vi "Hysteresis-FromFwdBwdHoneyCombStructure.vi"(4 "Max Hysteresis":dbl=0.2 format="%#_13g", 6 "border filter":dbl format="%#_13g", 8 "hypothesis":T1(ring)=enum."middle", 9 "relative Range":dbl=0.5 min=0.0 max=1.0 format="%#_13g", 10 "Pictures":cluster{"Fwd":dbl[][], "Bwd":dbl[][]}) -> (0 "bwd_fwd_weight":cluster{dbl[], dbl[], dbl[]}, 1 "Preisach":dbl[](array[numeric]), 2 "Polynomial Coefficients bwd":dbl[](array[numeric]), 3 "Polynomial Coefficients fwd":dbl[](array[numeric]), 5 "pixel to delete":i32)   [LabVIEW 2016]
uses:
  <vilib>/Analysis/NI_AALPro.lvlib
panel:
  out "Cov processed":dbl[][](graph)
  out "Hysteresis loop":cluster{dbl[], dbl[]}[](graph)
  out "Cov unprocessed":dbl[][](graph)
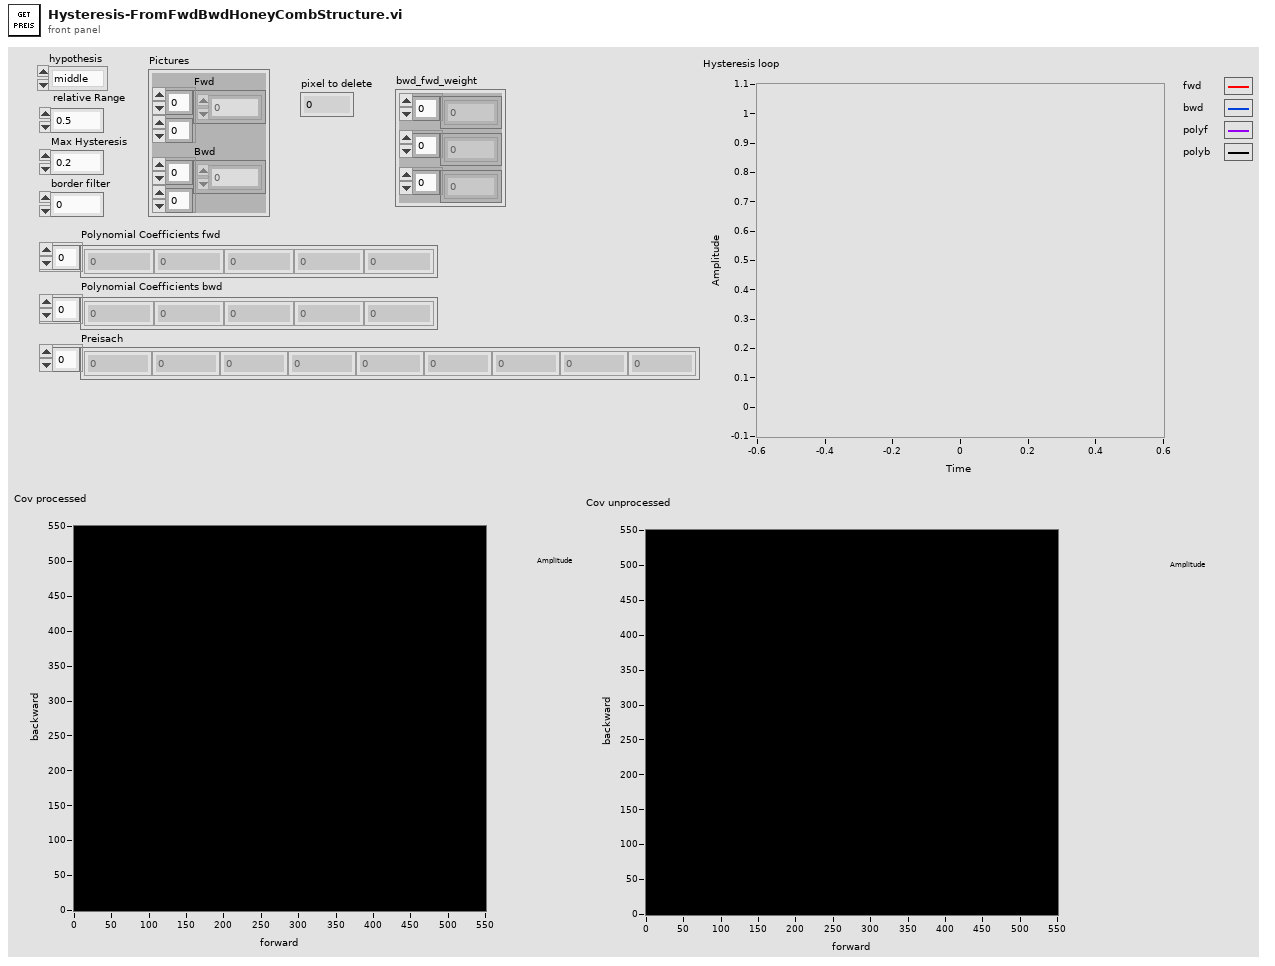
[diagram p1: front panel]
types:
  T1 = enum16{"bwd", "middle", "fwd", "linear", "2nd esti"}
  T2 = cluster{"bwd column corrected":dbl[], "fwd column corrected":dbl[]}
  T3 = cluster{"linear pos ":dbl[], "bwd pos":dbl[], "fwd pos":dbl[]}
  T4 = cluster{"bwd column corrected":dbl[], "fwd column corrected":dbl[], "Values":dbl[]}
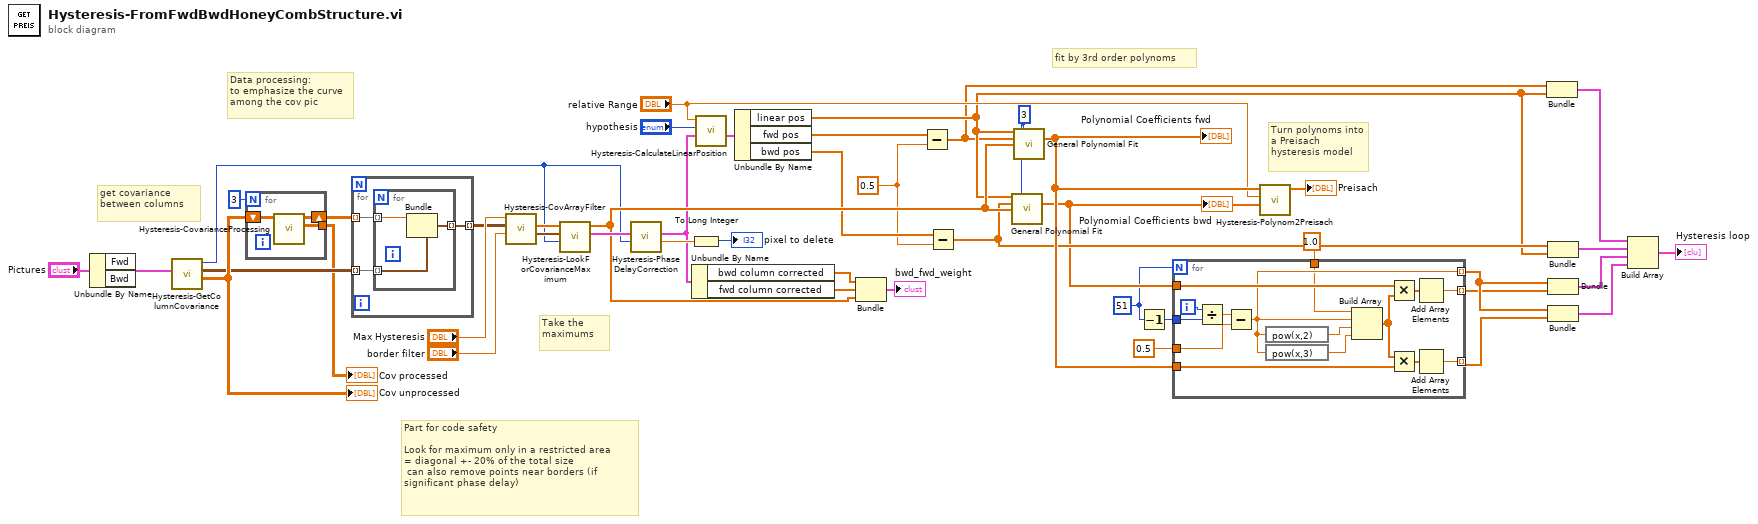
[diagram p0: block diagram]
diagram:
  w7 = 0.5 ("y")
  w4 = 3 ("polynomial order")
  w1 = 51
  # "Take the maximums"
  # "fit by 3rd order polynoms"
  # "Turn polynoms into a Preisach hysteresis model"
  # "Part for code safety\n\nLook for maximum only in a restricted area\n= diagonal +- 20% of the total size\n can also remove points near borders (if significant phase delay)"
  # "Data processing:\nto emphasize the curve\namong the cov pic"
  # "get covariance between columns"
  n1 = Unbundle By Name("Pictures") -> ()  [unwired: 2 out]
  n2 = call "Hysteresis-GetColumnCovariance.vi"("Pictures"="Pictures") -> ("Covariances (2D)"=w32:dbl[][], "Covariances (in cluster)"=w30:cluster{dbl, i32, i32}[][], "Size"=w20:i32)  [unwired: 8 in]
  "Cov unprocessed" <- w32
  n3 = for {
    N: 3 -> [_]
    tunnel: [w46] -> w3
    shift-right: [w47] -> w31
    shift-left: w32 -> [w48]
    n4 = call "Hysteresis-CovarianceProcessing.vi"("Covariances (2D)"=w48) -> ("Covariance Processed (2D)"=w46:dbl[][], "Covariance Data"=w47:dbl[][])  [unwired: 9 in]
  }
  "Cov processed" <- w3
  n5 = for {
    tunnel: w31 -> [w50] mode=indexing
    tunnel: w30 -> [w51] mode=indexing
    tunnel: [w49] -> w29 mode=indexing
    n6 = for {
      tunnel: w51 -> [w54] mode=indexing
      tunnel: w50 -> [w53] mode=indexing
      tunnel: [w52] -> w49 mode=indexing
      n7 = Bundle(cluster=w54, w53) -> (w52:cluster{dbl, i32, i32})  [unwired: 2 in]
    }
  }
  n8 = call "Hysteresis-CovArrayFilter.vi"("filtering"="border filter", "Covariance Corrected"=w29, "Max Hysteresis"="Max Hysteresis") -> ("Cluster filtered"=w41:cluster{dbl, i32, i32}[], "Covariance Values (1D)"=w42:dbl[])  [unwired: 7 in]
  n9 = call "Hysteresis-LookForCovarianceMaximum.vi"("size"=w20, "Cluster filtered"=w41, "Covariance Values (1D)"=w42) -> ("BWD/FWD"=w45:cluster{"bwd column":i32[], "fwd column":i32[]}, "Values"=w24:dbl[])  [unwired: 7 in]
  n10 = call "Hysteresis-PhaseDelayCorrection.vi"("size"=w20, "FWD/BWD"=w45) -> ("pixel to delete"=w26:dbl, "Corrected"=w9:T2)  [unwired: 8 in]
  n11 = To Long Integer(number=w26) -> (32bit integer=→"pixel to delete":i32)
  n12 = Unbundle By Name(w9) -> ("bwd column corrected"=w16:dbl[], "fwd column corrected"=w15:dbl[])
  n13 = call "Hysteresis-CalculateLinearPosition.vi"("BWD/FWD"=w9, "hypothesis"="hypothesis", "relative Range"="relative Range") -> ("LinBwdFwd"=w14:T3)  [unwired: 8 in]
  n14 = Unbundle By Name(w14) -> ("linear pos"=w10:dbl[], "fwd pos"=w13:dbl[], "bwd pos"=w12:dbl[])
  n15 = Bundle("bwd column corrected"=w16, "fwd column corrected"=w15, "Values"=w24) -> (→"bwd_fwd_weight":T4)  [unwired: 1 in]
  n16 = Subtract(x=w13, y=w7) -> (x-y=w8:dbl[])
  n17 = Subtract(x=w12, y=w7) -> (x-y=w22:dbl[])
  n18 = call <vilib>:"General Polynomial Fit.vi"("Y"=w10, "polynomial order"=w4, "X"=w22, "Weight"=w24) -> ("Polynomial Coefficients"=w5:dbl[])  [unwired: 8 in, 3 out]
  "Polynomial Coefficients bwd" <- w5
  n19 = call <vilib>:"General Polynomial Fit.vi"("Y"=w10, "polynomial order"=w4, "X"=w8, "Weight"=w24) -> ("Polynomial Coefficients"=w25:dbl[])  [unwired: 8 in, 3 out]
  "Polynomial Coefficients fwd" <- w25
  n20 = Decrement(x=w1) -> (x-1=w11:i32)
  n21 = for {
    N: w1 -> [_]
    tunnel: w5 -> [w67]
    tunnel: w25 -> [w61]
    tunnel: [w64] -> w35 mode=indexing
    tunnel: [w60] -> w34 mode=indexing
    tunnel: [w57] -> w36 mode=indexing
    tunnel: w11 -> [w62]
    tunnel: 0.5 ("y") -> [w56]
    tunnel: 1.0 -> [w55]
    i -> [w69]
    n22 = Divide(x=w69, y=w62) -> (x/y=w63:dbl)
    n23 = Subtract(x=w63, y=w56) -> (x-y=w57:dbl)
    n24 = expression code="pow(x,2)"(w57) -> (w59:dbl)
    n25 = expression code="pow(x,3)"(w57) -> (w58:dbl)
    n26 = Build Array(w55, w57, w59, w58) -> (w68:dbl[])
    n27 = Multiply(x=w67, y=w68) -> (x*y=w65:dbl[])
    n28 = Multiply(x=w68, y=w61) -> (x*y=w66:dbl[])
    n29 = Add Array Elements(numeric array=w65) -> (sum=w64:dbl)
    n30 = Add Array Elements(numeric array=w66) -> (sum=w60:dbl)
  }
  n31 = call "Hysteresis-Polynom2Preisach.vi"("Polynomial Coefficients bwd"=w5, "relative Range"="relative Range", "Polynomial Coefficients fwd"=w25) -> ("Preisach"=→"Preisach":dbl[])  [unwired: 8 in]
  n32 = Bundle(w8, "linear pos"=w10) -> (w27:cluster{dbl[], "linear pos ":dbl[]})  [unwired: 1 in]
  n33 = Bundle(w22, "linear pos"=w10) -> (w28:cluster{dbl[], "linear pos ":dbl[]})  [unwired: 1 in]
  n34 = Bundle(w36, w35) -> (w38:cluster{dbl[], dbl[]})  [unwired: 1 in]
  n35 = Bundle(w36, w34) -> (w37:cluster{dbl[], dbl[]})  [unwired: 1 in]
  n36 = Build Array(w27, w28, w38, w37) -> (→"Hysteresis loop":cluster{dbl[], "linear pos ":dbl[]}[])
